vi "Highligth Selected Row.vi"(8 "error in":errorcluster, 9 "Current Row":i32, 11 "Table in":refnum<vi>) -> (0 "error out":errorcluster)   [LabVIEW 2025, in "Automotive Ethernet Bus Monitor UI.lvlib"]
doc: "Set currently selected row as the highlighted one, and remove the highligth from the previous one."
uses:
  Automotive Ethernet Bus Monitor UI.lvlib
  <vilib>/Utility/miscctls.llb/LVRowAndColumnTypeDef.ctl
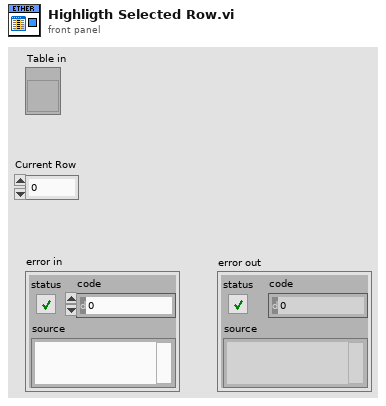
[diagram p1: front panel]
types:
  T1 = typedef "LVRowAndColumnTypeDef.ctl" = cluster{"Row":i32, "Column":i32}
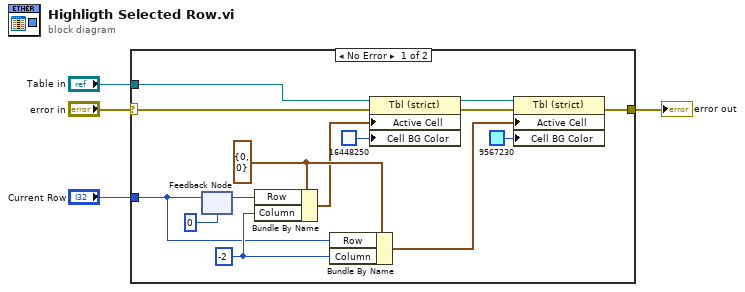
[diagram p0: block diagram]
diagram:
  n1 = case shown="No Error" "error in" {
    selector: "error in" -> [w6 w19]
    tunnel: [w18 w19] -> w4
    tunnel: "Table in" -> [w15 _]
    tunnel: "Current Row" -> [w5 _]
    frame No Error {
      w13 = -2 ("Column")
      w14 = T1 {"Row"=0, "Column"=0} ("Active Cell:Active Cell")
      n2 = feedback #1(0 ("Row")) -> (w10:i32)
      n3 = feedback-in #1(w5) -> ()
      n4 = Bundle By Name(cluster=w14, "Row"=w10, "Column"=w13) -> (w12:T1)
      n5 = Bundle By Name(cluster=w14, "Row"=w5, "Column"=w13) -> (w9:T1)
      n6 = property class="Tbl (strict)"(reference=w15, error in=w6, "Active Cell"=w12, "Cell BG Color"=u32 16448250 ("Active Cell:Cell Background Color")) -> (reference out=w16:refnum<vi>, error out=w17:errorcluster)
      n7 = property class="Tbl (strict)"(reference=w16, error in=w17, "Active Cell"=w9, "Cell BG Color"=u32 9567230 ("Active Cell:Cell Background Color")) -> (error out=w18:errorcluster)  [unwired: 1 out]
    }
    frame Error {
    }
  }
  "error out" <- w4
